vi "Send autofocus info.vi"(8 "error in (no error)":errorcluster, 11 "Tomo in":refnum<class "Tomo.lvclass">) -> (0 "error out":errorcluster, 3 "Tomo out":refnum<class "Tomo.lvclass">)   [LabVIEW 2012, in "Tomo.lvclass"]
uses:
  Tomo.lvclass
  <vilib>/Distrio/Murmex/Murmex/Murmex.lvclass
  <vilib>/Distrio/Murmex/Murmex/update_cluster.ctl
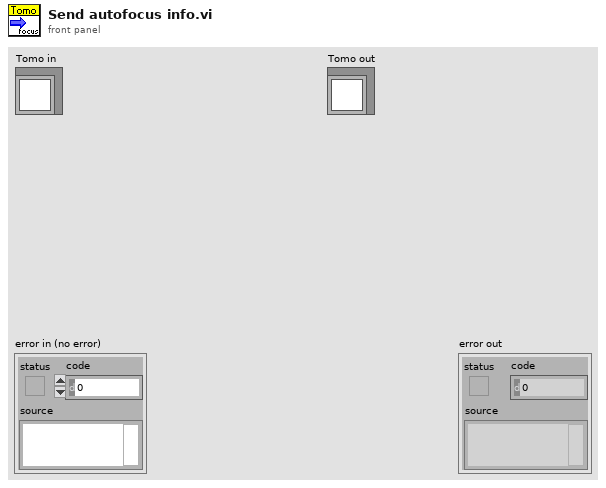
[diagram p1: front panel]
types:
  T1 = typedef "Murmex.lvlib/Murmex.lvclass/update_cluster.ctl" = cluster{"target ID":string, "key chains":string[], "values":variant[]}
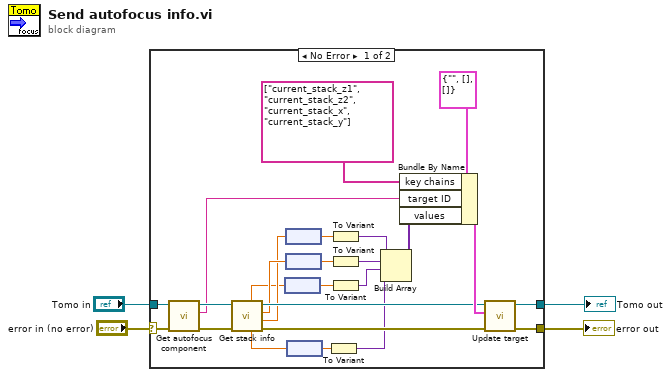
[diagram p0: block diagram]
diagram:
  n1 = case shown="No Error" "error in (no error)" {
    selector: "error in (no error)" -> [w20 w31]
    tunnel: [w24 w31] -> w3
    tunnel: [w26 w30] -> w2
    tunnel: "Tomo in" -> [w22 w30]
    frame No Error {
      n2 = call-dynamic "Get autofocus component.vi"("error in (no error)"=w20, "Tomo in"=w22) -> ("error out"=w19:errorcluster, "autofocus component"=w18:string, "Tomo out"=w21:refnum<class "Tomo.lvclass">)  [unwired: 7 in]
      n3 = call-dynamic "Get stack info.vi"("error in (no error)"=w19, "Tomo in"=w21) -> ("error out"=w25:errorcluster, "Z start"=w16:dbl, "Z stop"=w17:dbl, "Tomo out"=w27:refnum<class "Tomo.lvclass">, "Y position"=w9:dbl, "X position"=w10:dbl)  [unwired: 4 in]
      n4 = node(w10) -> (w8:dbl[unit])
      n5 = node(w16) -> (w15:dbl[unit])
      n6 = node(w17) -> (w14:dbl[unit])
      n7 = node(w9) -> (w7:dbl[unit])
      n8 = To Variant(anything=w7) -> (Variant=w5:variant)
      n9 = To Variant(anything=w15) -> (Variant=w13:variant)
      n10 = To Variant(anything=w14) -> (Variant=w12:variant)
      n11 = To Variant(anything=w8) -> (Variant=w6:variant)
      n12 = Build Array(w13, w12, w6, w5) -> (w11:variant[])
      n13 = Bundle By Name(cluster=T1 {"target ID"="", "key chains"=[], "values"=[]} ("update cluster"), "key chains"=string[] ["current_stack_z1", "current_stack_z2", "current_stack_x", "current_stack_y"], "target ID"=w18, "values"=w11) -> (w29:T1)
      n14 = call <vilib>:"Update target.vi"("error in (no error)"=w25, "update cluster"=w29, "MurmexBase in"=w27) -> ("error out"=w24:errorcluster, "MurmexBase out"=w26:refnum<class "Tomo.lvclass">)  [unwired: 7 in]
    }
    frame Error {
    }
  }
  "error out" <- w3
  "Tomo out" <- w2
